vi "task8.vi"() -> ()   [LabVIEW 2017]
panel:
  out "Value:":string
  in  "Select number system":T1(radio)
  in  "Boolean 7":bool
  in  "Boolean 6":bool
  in  "Boolean 5":bool
  in  "Boolean 4":bool
  in  "Boolean 3":bool
  in  "Boolean 2":bool
  in  "Boolean":bool
  in  "Boolean":bool
  in  "stop":bool
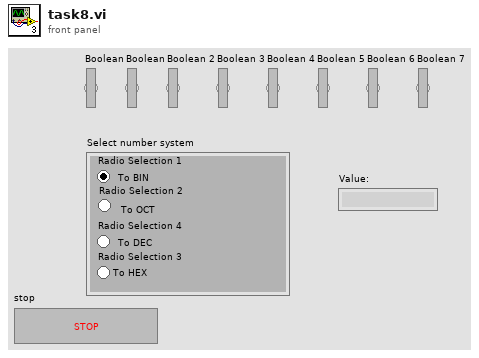
[diagram p1: front panel]
types:
  T1 = enum32{"Radio Selection 1", "Radio Selection 2", "Radio Selection 3", "Radio Selection 4"}
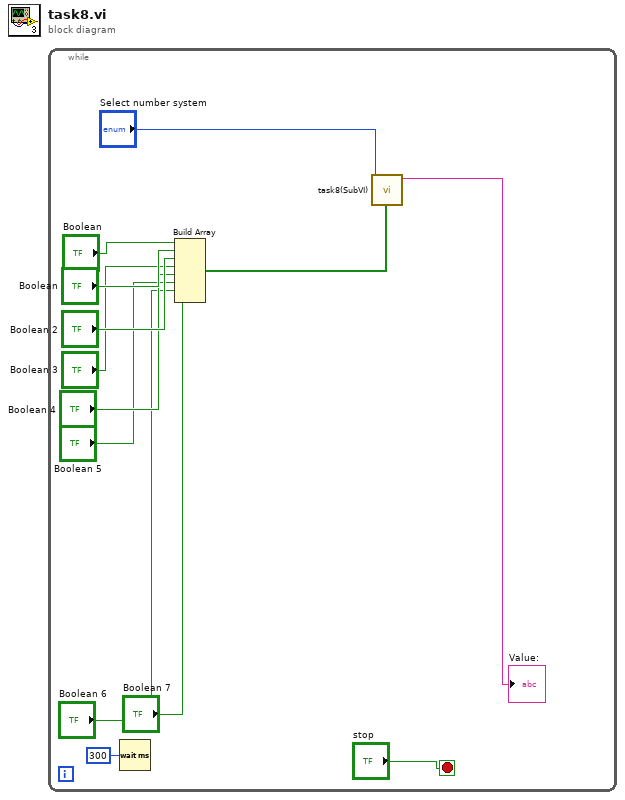
[diagram p0: block diagram]
diagram:
  n1 = while {
    stop <- "stop" stop-if-true
    n2 = Wait (ms)(milliseconds to wait=u32 300) -> ()  [unwired: 1 out]
    n3 = Build Array("Boolean", "Boolean", "Boolean 2", "Boolean 3", "Boolean 4", "Boolean 5", "Boolean 6", "Boolean 7") -> (w3:bool[])
    n4 = call "task8(SubVI).vi"("Array"=w3, "Select number system"="Select number system") -> ("Value:"=→"Value:":string)  [unwired: 9 in]
  }
